vi "ShooterMain.vi"(7 "Manual Input":dbl, 8 "Error In":errorcluster, 9 "Current RPM":dbl, 10 "Target RPM":dbl, 11 "Mode":enum16{"Open", "PID Control", "Manual Control"}(ring)) -> (0 "Error Out":errorcluster, 2 "Output":dbl)   [LabVIEW 2016]
uses:
  <vilib>/Rock Robotics/SystemInterfaces/DIO/FPGA_DIOPWMChannel.ctl
  <vilib>/Rock Robotics/WPI/MotorControl/WPI_MotorControlOpen VictorSP.vi
  <vilib>/addons/control/pid/pid.llb/PID (DBL).vi
  <vilib>/addons/control/pid/NI_PID_pid.lvlib
panel:
  in  "PID gains":T1={"proportional gain (Kc)"=1.0, "integral time (Ti, min)"=0.01, "derivative time (Td, min)"=0.0} {"derivative time (Td, min)" format="%.3f"; "integral time (Ti, min)" format="%.3f"; "proportional gain (Kc)" format="%.3f"}
  # "2017 Shooter Main Control VI\nFRC Team 34"
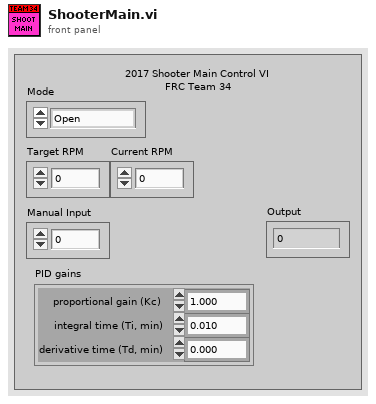
[diagram p1: front panel]
types:
  T1 = cluster{"proportional gain (Kc)":dbl, "integral time (Ti, min)":dbl, "derivative time (Td, min)":dbl}
  T2 = typedef "FPGA_DIOPWMChannel.ctl" = enum8{"PWM 0", "PWM 1", "PWM 2", "PWM 3", "PWM 4", "PWM 5", "PWM 6", "PWM 7", "PWM 8", "PWM 9", "PWM MXP 0", "PWM MXP 1", "PWM MXP 2", "PWM MXP 3", "PWM MXP 4", "PWM MXP 5", "PWM MXP 6", "PWM MXP 7", "PWM MXP 8", "PWM MXP 9", "Invalid"}
  T3 = typedef "WPI_MotorControlDeviceRef.ctl" = cluster{"DeviceStatus":errorcluster, "Type":T4, "PWM":cluster{"PWM Channel":T2, "DeadBand":T5}, "CAN":cluster{"Device Number":u8, "SetOutput VI Ref":variant, "GetOutput VI Ref":variant, "Enable VI Ref":variant, "Disable VI Ref":variant, "Data":variant}, "Invert":bool}
  T4 = typedef "WPI_MotorControlType.ctl" = enum16{"PWM", "CAN"}
  T5 = typedef "WPI_PWMDeadband.ctl" = cluster{"Name":string, "maxPositivePwm":i32, "minPositivePwm":i32, "centerPwm":i32, "maxNegativePwm":i32, "minNegativePwm":i32, "angularRange":u16}
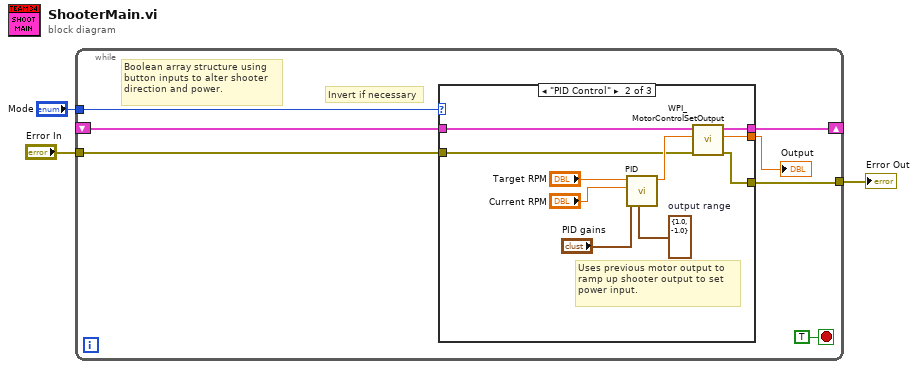
[diagram p0: block diagram]
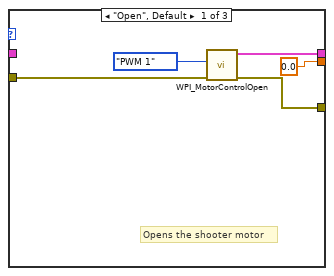
[diagram p2: hidden frame]
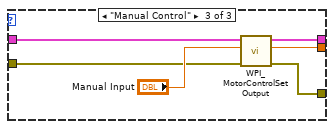
[diagram p3: hidden frame]
diagram:
  n1 = while {
    tunnel: "Mode" -> [w9]
    shift-right: [w8] -> _
    shift-left: _ -> [w7]
    tunnel: "Error In" -> [w5]
    tunnel: [w4] -> w1
    stop <- TRUE stop-if-true
    # "Invert if necessary"
    # "Boolean array structure using \nbutton inputs to alter shooter\ndirection and power."
    n2 = case shown="\"PID Control\"" w9 {
      tunnel: [w15 w24 w30] -> w8
      tunnel: w7 -> [_ w25 w31]
      tunnel: [0.0 ("Motor Output") w23 w29] -> w6
      tunnel: w5 -> [w12 w17 w27]
      tunnel: [w11 w16 w26] -> w4
      frame "Open", Default {
        # "Opens the shooter motor"
        n3 = call-poly <vilib>:"WPI_MotorControlOpen.vi"("error in (no error)"=w12, "PWM Channel"=FPGA_DIOPWMChannel."PWM 1") -> ("error out"=w11:errorcluster, "MotorControlDeviceRef"=w15:T3)  [unwired: 8 in]
      }
      frame "PID Control" {
        w20 = cluster{"output high":dbl, "output low":dbl} {"output high"=1.0, "output low"=-1.0}  # output range
        # "Uses previous motor output to\nramp up shooter output to set\npower input."
        n4 = call-poly <vilib>:"PID.vi"("output range"=w20, "PID gains"="PID gains", "process variable"="Current RPM", "setpoint"="Target RPM") -> ("output"=w18:dbl)  [unwired: 6 in, 1 out]
        n5 = call <vilib>:"WPI_MotorControlSetOutput.vi"("error in (no error)"=w17, "Output"=w18, "MotorControlDevRef"=w25) -> ("error out"=w16:errorcluster, "Motor Output"=w23:dbl, "MotorControlDevRef"=w24:T3)  [unwired: 6 in]
      }
      frame "Manual Control" {
        n6 = call <vilib>:"WPI_MotorControlSetOutput.vi"("error in (no error)"=w27, "Output"="Manual Input", "MotorControlDevRef"=w31) -> ("error out"=w26:errorcluster, "Motor Output"=w29:dbl, "MotorControlDevRef"=w30:T3)  [unwired: 6 in]
      }
    }
    "Output" <- w6
  }
  "Error Out" <- w1
